vi "Write Message.vi"(7 "Message Type":T1, 8 "timeout ms (5000)":i32=5000, 9 "Message":u8[](array[numeric]), 10 "error in (no error)":errorcluster, 11 "RawSocket Handler in":refnum<class "RawSocket TCP Handler.lvclass">) -> (2 "error out":errorcluster, 3 "RawSocket Handler out":refnum<class "RawSocket TCP Handler.lvclass">)   [LabVIEW 2020, in "wamplv.lvlib" / "RawSocket TCP Handler.lvclass"]
uses:
  RawSocket TCP Handler.lvclass
  TypeDefs/Message Type.ctl
  RawSocket TCP Handler.lvclass/RawSocket TCP Handler.ctl
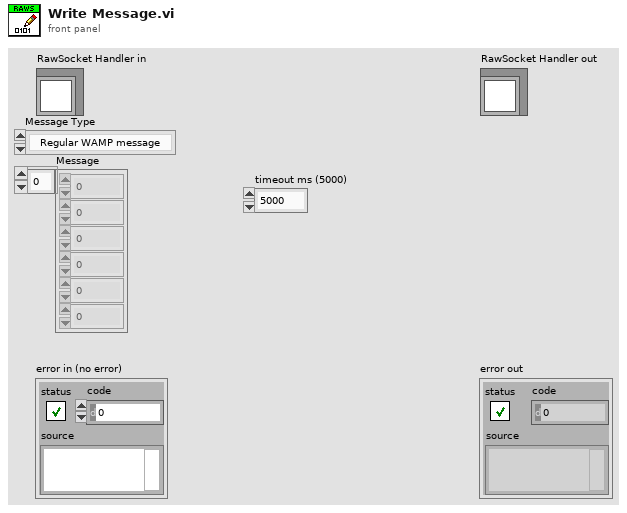
[diagram p1: front panel]
types:
  T1 = typedef "wamplv.lvlib/RawSocket TCP Handler.lvclass/Message Type.ctl" = enum8{"Regular WAMP message", "PING", "PONG"}
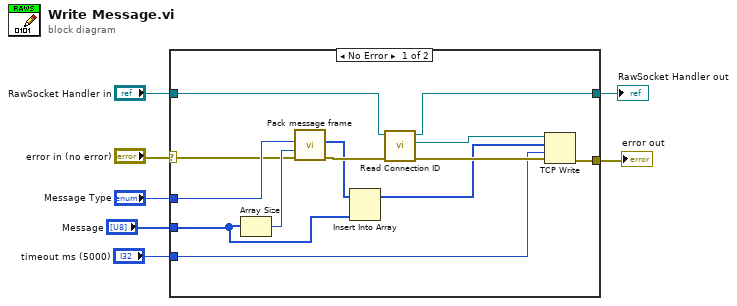
[diagram p0: block diagram]
diagram:
  n1 = case shown="No Error" "error in (no error)" {
    selector: "error in (no error)" -> [w16 w21]
    tunnel: "Message Type" -> [w20 _]
    tunnel: "RawSocket Handler in" -> [w15 w22]
    tunnel: [w14 w22] -> w4
    tunnel: "timeout ms (5000)" -> [w12 _]
    tunnel: [w11 w21] -> w2
    tunnel: "Message" -> [w8 _]
    frame No Error {
      n2 = Array Size(array=w8) -> (size(s)=w19:i32)
      n3 = call "Pack message frame.vi"("error in"=w16, "Size (bytes)"=w19, "Message Type"=w20) -> ("error out"=w18:errorcluster, "Message frame"=w10:u8[])  [unwired: 7 in]
      n4 = Insert Into Array(array=w10, new element=w8) -> (w9:u8[])  [unwired: 1 in]
      n5 = call-dynamic "Read Connection ID.vi"("error in (no error)"=w18, "RawSocket Handler in"=w15) -> ("error out"=w17:errorcluster, "Connection ID"=w13:refnum<k5>, "RawSocket Handler out"=w14:refnum<class "RawSocket TCP Handler.lvclass">)  [unwired: 7 in]
      n6 = TCP Write(connection ID=w13, data in=w9, error in (no error)=w17, 9:w12) -> (error out=w11:errorcluster)  [unwired: 2 out]
    }
    frame Error {
    }
  }
  "error out" <- w2
  "RawSocket Handler out" <- w4
